vi "Get Components Target Directory.vi"(8 "error in (no error)":errorcluster, 11 "Item Ref in":T1 format="%.0x") -> (0 "error out":errorcluster, 2 "components target directory":path, 3 "Item Ref out":T1 format="%.0x")   [LabVIEW 2017, in "DSF Shared.lvlib"]
uses:
  DSF Shared.lvlib
  <vilib>/NI Veristand/Custom Device API/Custom Device Item Ref.ctl
  <vilib>/NI Veristand/Custom Device API/Get Item Property (Path).vi
  <vilib>/NI Veristand/Custom Device API/Custom Device API.lvlib
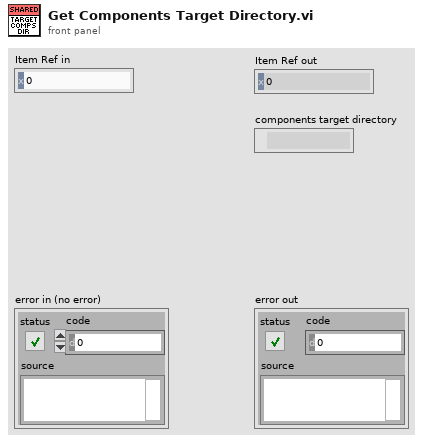
[diagram p1: front panel]
types:
  T1 = typedef "Custom Device API.lvlib/Custom Device Item Ref.ctl" = u64
  T2 = typedef "Custom Device API.lvlib/Custom Device Target Type.ctl" = enum16{"PharLap", "VxWorks", "Windows", "Linux_32_ARM", "Linux_x64"}
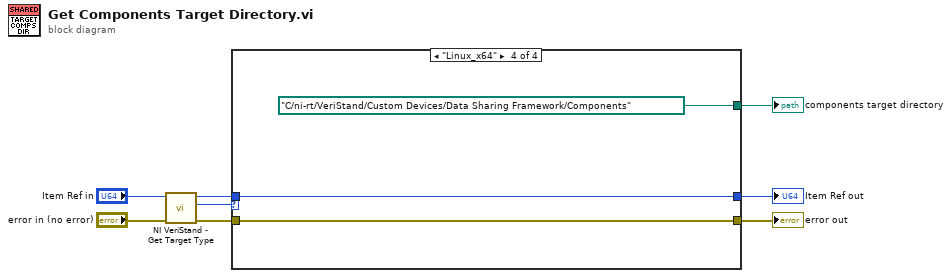
[diagram p0: block diagram]
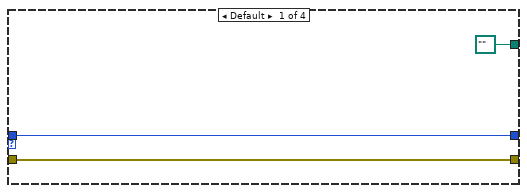
[diagram p2: hidden frame]
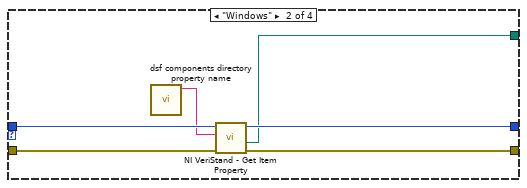
[diagram p3: hidden frame]
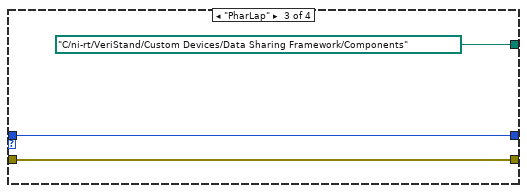
[diagram p4: hidden frame]
diagram:
  n1 = call <vilib>:"NI VeriStand - Get Target Type.vi"("error in (no error)"="error in (no error)", "Item Ref in"="Item Ref in") -> ("error out"=w4:errorcluster, "Target Type"=w6:T2, "Item Ref out"=w5:T1)  [unwired: 7 in]
  n2 = case shown="\"Linux_x64\"" w6 {
    tunnel: w5 -> [w11 w17 w19 w22]
    tunnel: w4 -> [w10 w16 w20 w23]
    tunnel: [path "" ("appended path") w13 path "C:/ni-rt/VeriStand/Custom Devices/Data Sharing Framework/Components" ("RT Destination") path "C:/ni-rt/VeriStand/Custom Devices/Data Sharing Framework/Components" ("RT Destination")] -> w3
    tunnel: [w10 w14 w20 w23] -> w2
    tunnel: [w11 w15 w19 w22] -> w1
    frame Default {
    }
    frame "Windows" {
      n3 = call "dsf components directory property name.vi"() -> ("components directory property name"=w12:string)  [unwired: 11 in]
      n4 = call-poly <vilib>:"NI VeriStand - Get Item Property.vi"("error in (no error)"=w16, "Property Name"=w12, "Item Ref in"=w17) -> ("error out"=w14:errorcluster, "Value"=w13:path, "Item Ref out"=w15:T1)  [unwired: 5 in, 1 out]
    }
    frame "PharLap" {
    }
    frame "Linux_x64" {
    }
  }
  "Item Ref out" <- w1
  "error out" <- w2
  "components target directory" <- w3
